vi "Relaunch uService.vi"(8 "error in (no error)":errorcluster, 9 "uService Properties":T1, 10 "uService ID":string, 11 "Guardian in":refnum<class "Guardian.lvclass">) -> (0 "error out":errorcluster, 3 "Guardian out":refnum<class "Guardian.lvclass">)   [LabVIEW 2026, in "TALOS.lvlib" / "Guardian.lvlib" / "Guardian.lvclass"]
doc: "SubVI of Handle Last Ack Core: check if the uService that has just died needs to be restarted, and in case it does."
uses:
  Guardian.lvclass
  C:/LabVIEW Code/TALOS/builds/Actor Framework PPL/Actor Framework.lvlibp/1abvi3w/vi.lib/ActorFramework/Actor/Actor.lvclass
  Classes/uService List/uService Properties.ctl
  builds/Actor Framework PPL/Actor Framework.lvlibp/1abvi3w/vi.lib/ActorFramework/Message Enqueuer/Message Enqueuer.lvclass
  Guardian.lvclass/Guardian.ctl
  Guardian Messages/Launch uService Msg/Launch uService Msg.lvclass/Launch uService Msg.ctl
  Ancestor/Ancestor/Ancestor.lvclass/Ancestor.ctl
  a147f722-f81d-4630-a913-877bdb8ea9c7.vi
  fad1abe8-d4a9-4cc8-99f2-89479e492748.vi
  Support VIs/Generate Error.vi
  FGV/Error Memory/Get Error Description.vi
  Support VIs/Get PC name.vi
  Ancestor/Ancestor/Read ID.vi
  Support VIs/Get Class Name.vi
  <vilib>/Utility/error.llb/Clear Errors.vi
  FGV/Error Memory/Error Memory Core.vi
  <vilib>/AdvancedString/Delimited String to 1D String Array.vi
  <vilib>/AdvancedString/Delimited String to 1D String Array (string).vi
  Support VIs/Circus Root Path.vi
  FGV/Error Memory/Error Crt Lvl checker.vi
  FGV/Error Memory/Error Memory Core.vi/40c8088d-b597-4017-91af-faa98e00292e.vi
  FGV/Error Memory/Error Memory Core.vi/d4a3ab98-063c-4e44-b43d-fbdcfe6c2be2.vi
  builds/Actor Framework PPL/Actor Framework.lvlibp/1abvi3w/vi.lib/ActorFramework/Message Enqueuer/Enqueue.vi
  Support VIs/Global Memory.vi
  <vilib>/Utility/LVClass/Get LV Class Name.vi
  Support VIs/Is in Packed Library.vi
  Support VIs/TALOS Root path.vi
  Support VIs/Read CSV worksheet.vi
  Support VIs/Global Constants.vi
  <vilib>/Utility/error.llb/General Error Handler.vi
  Support VIs/Error Log.vi
  <vilib>/Comparison/Equal/Equal Functor/Equal Functor.lvclass
  Guardian Messages/Launch uService Msg/Launch uService Msg.lvclass
  Ancestor/Ancestor/Ancestor.lvclass
  builds/Actor Framework PPL/Actor Framework.lvlibp/1abvi3w/vi.lib/ActorFramework/Actor/Actor.lvclass
  TALOS.lvlib
  Classes/uService List/uService List.lvclass
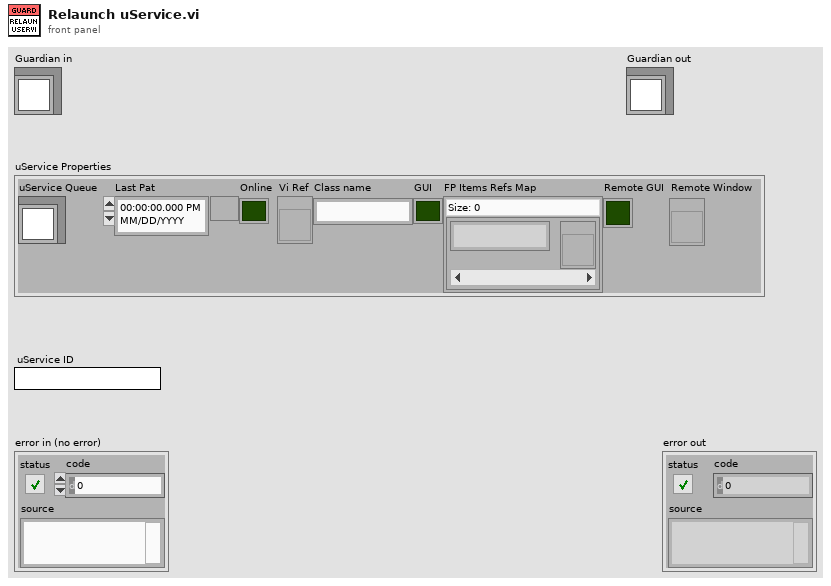
[diagram p1: front panel]
types:
  T1 = typedef "TALOS.lvlib/Classes.lvlib/uService List.lvclass/uService Properties.ctl" = cluster{"uService Queue":refnum<class "Message Enqueuer.lvclass">, "Last Pat":timestamp, "Online":bool, "Vi Ref":refnum<vi>, "Class name":string, "GUI":bool, "FP Items Refs Map":map{string, refnum<vi>}, "Remote GUI":bool, "Remote Window":refnum<vi>}
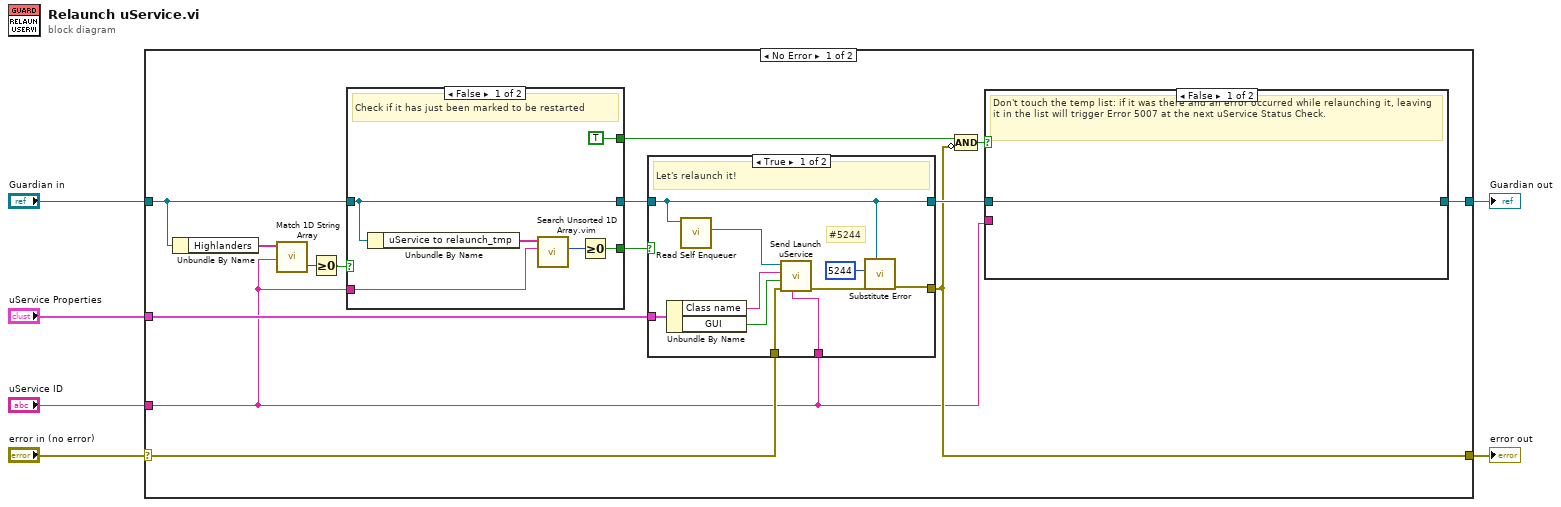
[diagram p0: block diagram]
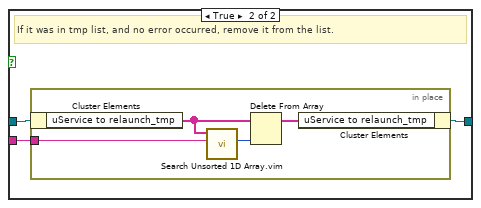
[diagram p2: hidden frame]
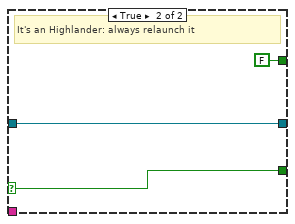
[diagram p3: hidden frame]
diagram:
  n1 = case shown="No Error" "error in (no error)" {
    selector: "error in (no error)" -> [w16 w50]
    tunnel: "Guardian in" -> [w20 w51]
    tunnel: "uService Properties" -> [w17 _]
    tunnel: [w12 w51] -> w3
    tunnel: [w11 w50] -> w2
    tunnel: "uService ID" -> [w9 _]
    frame No Error {
      n2 = Unbundle By Name(w20) -> ("Highlanders"=w10:string[])
      n3 = call <vilib>:"Match 1D String Array.vi"("Pattern"=w9, "Strings"=w10) -> ("index of element"=w8:i32)  [unwired: 2 in, 1 out]
      n4 = Greater Or Equal To 0?(x=w8) -> (x >= 0?=w7:bool)
      n5 = case shown="False" w7 {
        selector: w7 -> [_ w37]
        tunnel: w20 -> [w30 w36]
        tunnel: [w31 w37] -> w19
        tunnel: w9 -> [w33 _]
        tunnel: [w30 w36] -> w18
        tunnel: [TRUE FALSE] -> w15
        frame False {
          # "Check if it has just been marked to be restarted"
          n6 = Unbundle By Name(w30) -> ("uService to relaunch_tmp"=w34:string[])
          n7 = call "Search Unsorted 1D Array.vim"("element"=w33, "unsorted 1D array"=w34) -> ("index of element"=w32:i32)  [unwired: 9 in]
          n8 = Greater Or Equal To 0?(x=w32) -> (x >= 0?=w31:bool)
        }
        frame True {
          # "It's an Highlander: always relaunch it"
        }
      }
      n9 = case shown="True" w19 {
        tunnel: [w39 w49] -> w11
        tunnel: w18 -> [w38 w48]
        tunnel: w9 -> [w42 _]
        tunnel: w17 -> [w44 _]
        tunnel: w16 -> [w43 w49]
        tunnel: [w38 w48] -> w14
        frame True {
          # "#5244"
          # "Let's relaunch it!"
          n10 = Unbundle By Name(w44) -> ("Class name"=w47:string, "GUI"=w46:bool)
          n11 = call "Read Self Enqueuer.vi"("Actor"=w38) -> ("Self Enqueuer"=w45:refnum<class "Message Enqueuer.lvclass">)  [unwired: 10 in]
          n12 = call "Send Launch uService.vi"("uService ID"=w42, "error in (no error)"=w43, "GUI?"=w46, "uService Class Name"=w47, "Message Enqueuer"=w45) -> ("error out"=w40:errorcluster)  [unwired: 5 in, 1 out]
          n13 = call "Substitute Error.vi"("LabVIEW Object"=w38, "error in (no error)"=w40, "Error Code"=5244) -> ("error out"=w39:errorcluster)  [unwired: 8 in]
        }
        frame False {
          # "Not on the list, correctly closed"
        }
      }
      n14 = Compound Arithmetic op=AND(w15, invert w11) -> (w13:bool)
      n15 = case shown="False" w13 {
        tunnel: w14 -> [w21 w24]
        tunnel: w9 -> [_ w23]
        tunnel: [w21 w22] -> w12
        frame False {
          # "Don't touch the temp list: if it was there and an error occurred while relaunching it, leaving it in the list will trigger Error 5007 at the next uService Status Check."
        }
        frame True {
          # "If it was in tmp list, and no error occurred, remove it from the list."
          n16 = in-place {
            in-place-border: w23 -> [w28]
            n17 = in-place-cluster #1(w24) -> ("uService to relaunch_tmp"=w27:string[])
            n18 = call "Search Unsorted 1D Array.vim"("element"=w28, "unsorted 1D array"=w27) -> ("index of element"=w25:i32)  [unwired: 9 in]
            n19 = Delete From Array(array=w27, index=w25) -> (array with subset deleted=w26:string[])  [unwired: 1 in, 1 out]
            n20 = in-place-cluster #1("uService to relaunch_tmp"=w26) -> (w22:refnum<class "Guardian.lvclass">)
          }
        }
      }
    }
    frame Error {
    }
  }
  "error out" <- w2
  "Guardian out" <- w3
